vi "GetPulse4State.vi"(1 "PVD Board Cluster":T1[](array[typedef])=[{"DB Name"=0, "DB Delay (us)"=0, "DB Enabled"=TRUE, "Cap Name"=268}, {"DB Name"=1, "DB Delay (us)"=6, "DB Enabled"=TRUE, "Cap Name"=208}, {"DB Name"=2, "DB Delay (us)"=12, "DB Enabled"=TRUE, "Cap Name"=178}, {"DB Name"=3, "DB Delay (us)"=18, "DB Enabled"=TRUE, "Cap Name"=122}, {"DB Name"=4, "DB Delay (us)"=600, "DB Enabled"=TRUE, "Cap Name"=0}, {"DB Name"=5, "DB Delay (us)"=635, "DB Enabled"=TRUE, "Cap Name"=0}, {"DB Name"=6, "DB Delay (us)"=680, "DB Enabled"=TRUE, "Cap Name"=0}, {"DB Name"=7, "DB Delay (us)"=680, "DB Enabled"=TRUE, "Cap Name"=0}, {"DB Name"=8, "DB Delay (us)"=703, "DB Enabled"=TRUE, "Cap Name"=0}, {"DB Name"=9, "DB Delay (us)"=0, "DB Enabled"=FALSE, "Cap Name"=0}, {"DB Name"=10, "DB Delay (us)"=0, "DB Enabled"=FALSE, "Cap Name"=0}, {"DB Name"=11, "DB Delay (us)"=1000, "DB Enabled"=TRUE, "Cap Name"=0}, {"DB Name"=12, "DB Delay (us)"=0, "DB Enabled"=FALSE, "Cap Name"=0}, {"DB Name"=13, "DB Delay (us)"=0, "DB Enabled"=FALSE, "Cap Name"=0}, {"DB Name"=14, "DB Delay (us)"=0, "DB Enabled"=FALSE, "Cap Name"=0}, {"DB Name"=15, "DB Delay (us)"=65535, "DB Enabled"=FALSE, "Cap Name"=0}, {"DB Name"=16, "DB Delay (us)"=65535, "DB Enabled"=FALSE, "Cap Name"=0}, {"DB Name"=17, "DB Delay (us)"=65535, "DB Enabled"=FALSE, "Cap Name"=0}, {"DB Name"=18, "DB Delay (us)"=65535, "DB Enabled"=FALSE, "Cap Name"=0}, {"DB Name"=19, "DB Delay (us)"=65535, "DB Enabled"=FALSE, "Cap Name"=0}, {"DB Name"=20, "DB Delay (us)"=65535, "DB Enabled"=FALSE, "Cap Name"=0}, {"DB Name"=21, "DB Delay (us)"=65535, "DB Enabled"=FALSE, "Cap Name"=0}, {"DB Name"=22, "DB Delay (us)"=65535, "DB Enabled"=FALSE, "Cap Name"=0}, {"DB Name"=23, "DB Delay (us)"=65535, "DB Enabled"=FALSE, "Cap Name"=0}, {"DB Name"=24, "DB Delay (us)"=65535, "DB Enabled"=FALSE, "Cap Name"=0}, {"DB Name"=25, "DB Delay (us)"=65535, "DB Enabled"=FALSE, "Cap Name"=0}, {"DB Name"=26, "DB Delay (us)"=65535, "DB Enabled"=FALSE, "Cap Name"=0}, {"DB Name"=27, "DB Delay (us)"=65535, "DB Enabled"=FALSE, "Cap Name"=0}, {"DB Name"=28, "DB Delay (us)"=65535, "DB Enabled"=FALSE, "Cap Name"=0}, {"DB Name"=29, "DB Delay (us)"=65535, "DB Enabled"=FALSE, "Cap Name"=0}, {"DB Name"=30, "DB Delay (us)"=65535, "DB Enabled"=FALSE, "Cap Name"=0}, {"DB Name"=31, "DB Delay (us)"=65535, "DB Enabled"=FALSE, "Cap Name"=0}, {"DB Name"=32, "DB Delay (us)"=65535, "DB Enabled"=FALSE, "Cap Name"=0}, {"DB Name"=33, "DB Delay (us)"=65535, "DB Enabled"=FALSE, "Cap Name"=0}, {"DB Name"=34, "DB Delay (us)"=65535, "DB Enabled"=FALSE, "Cap Name"=0}, {"DB Name"=35, "DB Delay (us)"=65535, "DB Enabled"=FALSE, "Cap Name"=0}, {"DB Name"=36, "DB Delay (us)"=65535, "DB Enabled"=FALSE, "Cap Name"=0}, {"DB Name"=37, "DB Delay (us)"=65535, "DB Enabled"=FALSE, "Cap Name"=0}, {"DB Name"=38, "DB Delay (us)"=65535, "DB Enabled"=FALSE, "Cap Name"=0}, {"DB Name"=39, "DB Delay (us)"=65535, "DB Enabled"=FALSE, "Cap Name"=0}, {"DB Name"=40, "DB Delay (us)"=65535, "DB Enabled"=FALSE, "Cap Name"=0}, {"DB Name"=41, "DB Delay (us)"=65535, "DB Enabled"=FALSE, "Cap Name"=0}, {"DB Name"=42, "DB Delay (us)"=65535, "DB Enabled"=FALSE, "Cap Name"=0}, {"DB Name"=43, "DB Delay (us)"=65535, "DB Enabled"=FALSE, "Cap Name"=0}, {"DB Name"=44, "DB Delay (us)"=65535, "DB Enabled"=FALSE, "Cap Name"=0}, {"DB Name"=45, "DB Delay (us)"=65535, "DB Enabled"=FALSE, "Cap Name"=0}, {"DB Name"=46, "DB Delay (us)"=65535, "DB Enabled"=FALSE, "Cap Name"=0}, {"DB Name"=47, "DB Delay (us)"=65535, "DB Enabled"=FALSE, "Cap Name"=0}, {"DB Name"=48, "DB Delay (us)"=65535, "DB Enabled"=FALSE, "Cap Name"=0}, {"DB Name"=49, "DB Delay (us)"=65535, "DB Enabled"=FALSE, "Cap Name"=0}]) -> (0 "Pulse 4 Trigger Enabled":bool)   [LabVIEW 2016]
uses:
  CTControl/DBmanualControl.ctl
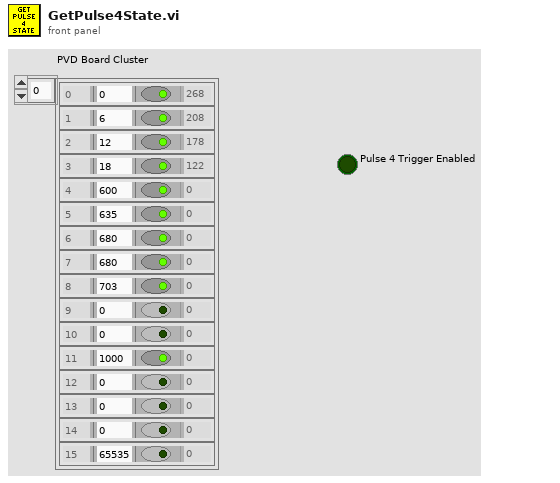
[diagram p1: front panel]
types:
  T1 = typedef "DBmanualControl.ctl" = cluster{"DB Name":u32, "DB Delay (us)":u32, "DB Enabled":bool, "Cap Name":u32}
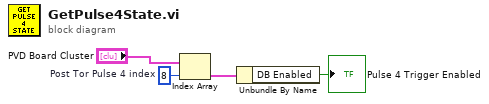
[diagram p0: block diagram]
diagram:
  w3 = 8  # Post Tor Pulse 4 index
  n1 = Index Array(array="PVD Board Cluster", index=w3) -> (element=w2:T1)
  n2 = Unbundle By Name(w2) -> ("DB Enabled"=→"Pulse 4 Trigger Enabled":bool)
